vi "Tags8bitgray_txt_res.vi"(0 "xbreite":u32, 1 "BigTiff":u8, 2 "yhöhe":u32, 3 "BildOffset Bytes":i64, 4 "Text length":u32, 5 "Text Offset Bytes":i64, 6 "Cluster":T1) -> (7 "Directory Entrys":T2[](array[typedef]))   [LabVIEW 2011]
uses:
  IFD.ctl
panel:
  # "bigtiff=1"
  # "Biftiff this is values!"
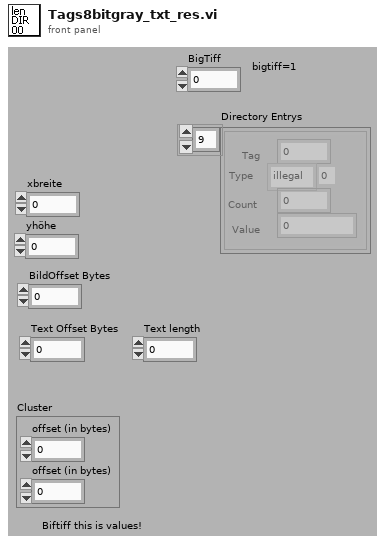
[diagram p1: front panel]
types:
  T1 = cluster{"offset (in bytes)":u64, "offset (in bytes)":u64}
  T2 = typedef "IFD.ctl" = cluster{"Tag":u16, "Type":enum16{"illegal", "Byte", "Ascii", "Short", "Long", "Rational", "SByte", "Undefined", "SShort", "SLong", "SRational 2xSLong", "Float 4byte", "Double 8Byte", "No13", "No14", "No15", "U64", "I64", "U64-IFD8"}, "Count":u64, "Value":u64}
  T3 = cluster{"Tag":u16, u16, "Count":u32, "Value":u32}
  T4 = enum16{"illegal", "Byte", "Ascii", "Short", "Long", "Rational", "SByte", "Undefined", "SShort", "SLong", "SRational 2xSLong", "Float 4byte", "Double 8Byte", "No13", "No14", "No15", "U64", "I64", "U64-IFD8"}
  T5 = cluster{"Width":u16, u16, "Count":u32, "xbreite":u32}
  T6 = cluster{"Lenght":u16, u16, "Count":u32, "yhöhe":u32}
  T7 = cluster{"ImageDescritionOffsets":u16, u16, "Text length":u32, "Text Offset Bytes":i64}
  T8 = cluster{"RowsPerStrip":u16, u16, "Count":u32, "yhöhe":u32}
  T9 = cluster{"StripOffsets":u16, "Type":enum16{"illegal", "Byte", "Ascii", "Short", "Long", "Rational", "SByte", "Undefined", "SShort", "SLong", "SRational 2xSLong", "Float 4byte", "Double 8Byte", "No13", "No14", "No15", "U64", "I64", "U64-IFD8"}, "Count":u32, "BildOffset Bytes":i64}
  T10 = cluster{"StripByteCount":u16, "Type":enum16{"illegal", "Byte", "Ascii", "Short", "Long", "Rational", "SByte", "Undefined", "SShort", "SLong", "SRational 2xSLong", "Float 4byte", "Double 8Byte", "No13", "No14", "No15", "U64", "I64", "U64-IFD8"}, "Count":u32, u64}
  T11 = cluster{"Xresolution":u16, u16, "Count":u32, "offset (in bytes)":u64}
  T12 = cluster{"yresolution":u16, u16, "Count":u32, "offset (in bytes)":u64}
  T13 = cluster{"resolutionunits":u16, u16, "Count":u32, "aribiträr":u32}
  T14 = cluster{"resolutionunits":u16, "Type":u16, "Count":u32, "offset (in bytes)":u64}[]
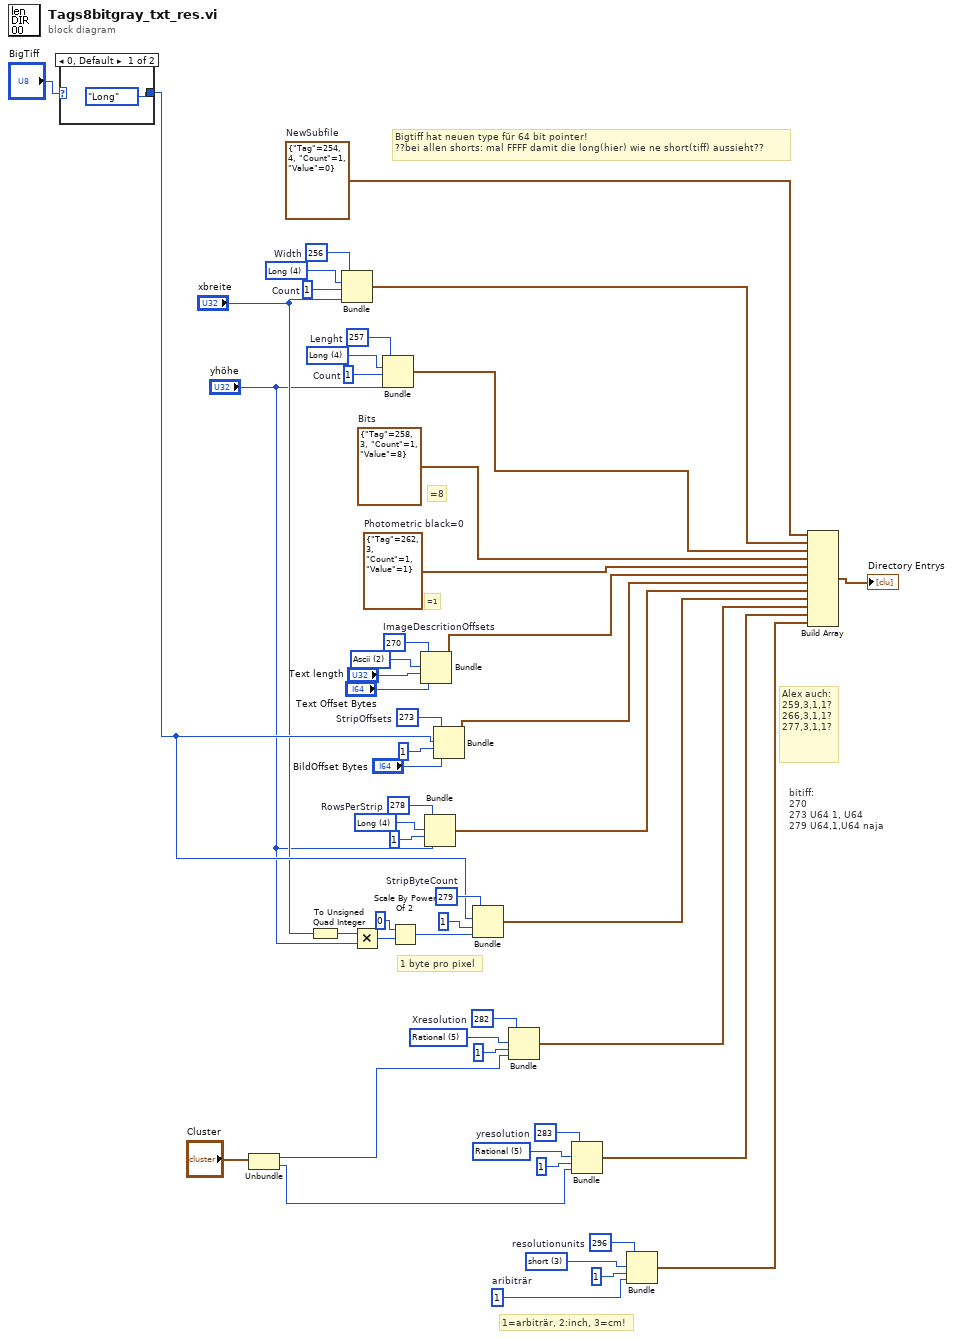
[diagram p0: block diagram]
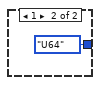
[diagram p2: hidden frame]
diagram:
  w7 = u32 1  # aribiträr
  w9 = u16 3 items=["illegal", "Byte", "Ascii", "short", "Long", "Rational", "SByte8", "Undefined", "SShort16", "SLong32", "SRational64", "Float32", "Double64"]
  w10 = u16 296  # resolutionunits
  w12 = u16 5 items=["illegal", "Byte", "Ascii", "short", "Long", "Rational", "SByte8", "Undefined", "SShort16", "SLong32", "SRational64", "Float32", "Double64"]
  w13 = u16 283  # yresolution
  w15 = u16 5 items=["illegal", "Byte", "Ascii", "short", "Long", "Rational", "SByte8", "Undefined", "SShort16", "SLong32", "SRational64", "Float32", "Double64"]
  w16 = u16 282  # Xresolution
  w23 = T3 {"Tag"=254, 4, "Count"=1, "Value"=0}  # NewSubfile
  w27 = u16 2 items=["illegal", "Byte", "Ascii", "short", "Long", "Rational"]
  w28 = u16 270  # ImageDescritionOffsets
  w33 = u16 273  # StripOffsets
  w43 = u16 279  # StripByteCount
  w45 = u16 4 items=["illegal", "Byte", "Ascii", "short", "Long", "Rational"]
  w46 = u16 278  # RowsPerStrip
  w36 = T3 {"Tag"=262, 3, "Count"=1, "Value"=1}  # Photometric black=0
  w47 = u16 4 items=["illegal", "Byte", "Ascii", "short", "Long", "Rational"]
  w48 = u32 1  # Count
  w49 = u16 257  # Lenght
  w50 = u16 4 items=["illegal", "Byte", "Ascii", "short", "Long", "Rational"]
  w51 = u32 1  # Count
  w52 = u16 256  # Width
  w37 = T3 {"Tag"=258, 3, "Count"=1, "Value"=8}  # Bits
  # "1=arbiträr, 2:inch, 3=cm!"
  # "1 byte pro pixel"
  # "Alex auch:\n259,3,1,1?\n266,3,1,1?\n277,3,1,1?"
  # "bitiff:\n270\n273 U64 1, U64\n279 U64,1,U64 naja"
  # "=1"
  # "=8"
  # "Bigtiff hat neuen type für 64 bit pointer!\n??bei allen shorts: mal FFFF damit die long(hier) wie ne short(tiff) aussieht??"
  n1 = case shown="0, Default" "BigTiff" {
    tunnel: [T4."Long" ("Type") T4."U64" ("Type")] -> w20
    frame 0, Default {
    }
    frame 1 {
    }
  }
  n2 = Unbundle("Cluster") -> ("offset (in bytes)"=w2:u64, "offset (in bytes)"=w1:u64)
  n3 = To Unsigned Quad Integer(1:"xbreite") -> (0:w17:u64)
  n4 = Bundle("Width"=w52, w50, "Count"=w51, "xbreite"="xbreite") -> (w24:T5)  [unwired: 1 out]
  n5 = Multiply(x=w17, y="yhöhe") -> (x*y=w40:u64)
  n6 = Bundle("Lenght"=w49, w47, "Count"=w48, "yhöhe"="yhöhe") -> (w38:T6)  [unwired: 1 out]
  n7 = Scale By Power Of 2(n=i16 0, x=w40) -> (x*2^n=w39:u64)
  n8 = Bundle("ImageDescritionOffsets"=w28, w27, "Text length"="Text length", "Text Offset Bytes"="Text Offset Bytes") -> (w22:T7)  [unwired: 1 out]
  n9 = Bundle("RowsPerStrip"=w46, w45, "Count"=u32 1, "yhöhe"="yhöhe") -> (w35:T8)  [unwired: 1 out]
  n10 = Bundle("StripOffsets"=w33, "Type"=w20, "Count"=u32 1, "BildOffset Bytes"="BildOffset Bytes") -> (w31:T9)  [unwired: 1 out]
  n11 = Bundle("StripByteCount"=w43, "Type"=w20, "Count"=u32 1, w39) -> (w34:T10)  [unwired: 1 out]
  n12 = Bundle("Xresolution"=w16, w15, "Count"=u32 1, "offset (in bytes)"=w2) -> (w6:T11)  [unwired: 1 out]
  n13 = Bundle("yresolution"=w13, w12, "Count"=u32 1, "offset (in bytes)"=w1) -> (w5:T12)  [unwired: 1 out]
  n14 = Bundle("resolutionunits"=w10, w9, "Count"=u32 1, "aribiträr"=w7) -> (w4:T13)  [unwired: 1 out]
  n15 = Build Array(w23, w24, w38, w37, w36, w22, w31, w35, w34, w6, w5, w4) -> (→"Directory Entrys":T14)
